vi "Set Amplitude.vi"(6 "Channel":i32=1, 8 "error in (no error)":errorcluster, 10 "Amplitude":dbl, 11 "336XX in":refnum<class "336XX.lvclass">) -> (0 "error out":errorcluster, 3 "336XX out":refnum<class "336XX.lvclass">)   [LabVIEW 2019, in "336XX.lvlib" / "336XX.lvclass"]
uses:
  Library/336XX.lvclass
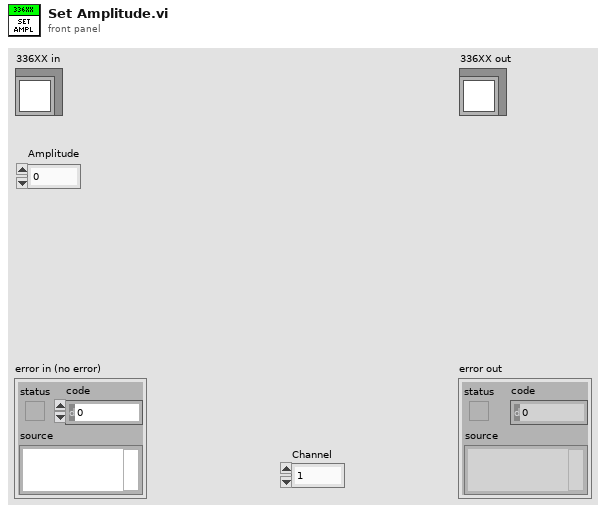
[diagram p1: front panel]
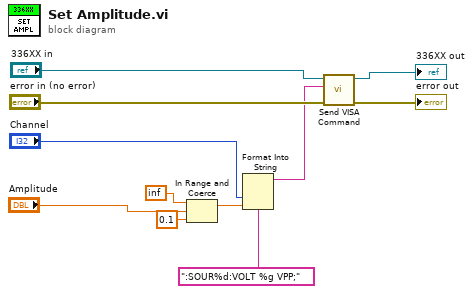
[diagram p0: block diagram]
diagram:
  n1 = In Range and Coerce(upper limit=inf, x="Amplitude", lower limit=0.1) -> (coerced(x)=w2:dbl)  [unwired: 1 out]
  n2 = Format Into String(format string=":SOUR%d:VOLT %g VPP;", "Channel", w2) -> (resulting string=w6:string)  [unwired: 2 in, 1 out]
  n3 = call "Send VISA Command.vi"("error in (no error)"="error in (no error)", "Command"=w6, "336XX in"="336XX in") -> ("error out"=→"error out":errorcluster, "336XX out"=→"336XX out":refnum<class "336XX.lvclass">)  [unwired: 7 in]
